vi "Meas Process Record.vi"(5 "result string label":string="str res", 7 "session":T9={"adc"={"niScope"={"channel cfg"=[], "sessions"=[], "multi cards"=FALSE, "channels"=0, "type"=enum."n/a", "memory [B/chn]"=0, "ext. clock [Hz]"=0.0, "samples count"=0, "use streaming"=FALSE, "proc setup"={"packet size [smpl]"=0, "current timeout [s]"=0.0, "blk2blk timeout [s]"=0.0, "event time"=timestamp(0 s since 1904-01-01), "temp sampl T [s]"=0.0, "data queue"=refnum, "stop notifier"=refnum, "proc ref"=refnum}, "sample width [B]"=0, "ranges [V]"=[], "trigger setup"={"coupling"=1, "level [V]"=0.0, "slope"=0, "mode"=enum."Immediate"}, "fs [Hz]"=0.0, "bitres [bit]"=0}, "3458A"={"channels"=[], "sync unit"={"VISA"="", "type"=enum."Picotest U6200A"}, "awg unit"={"type"=enum."Agilent 331xxA to 332xxA", "VISA"="", "enable 10MHz ref"=FALSE}, "sync mode"=enum."MASTER-SLAVE, MASTER clocked by TIMER", "streaming mode"=FALSE, "idn mode"=enum."Auto", "sampling mode"=enum."DCV", "Ts [s]"=0.0, "sample memory [B]"=0, "proc setup"={"channel id"=0, "packet size [smpl]"=0, "current timeout [s]"=0.0, "blk2blk timeout [s]"=0.0, "event time"=timestamp(0 s since 1904-01-01), "stop notifier"=refnum, "data queues"=[], "proc refs"=[], "bus semaphore"=refnum}, "sample size [B]"=0, "sample count"=0, "aux data"={"channel id"=0, "valid?"=[], "gain [V]"=[], "timestamp [s]"=[], "Ts [s]"=0.0, "abs timestamp"=timestamp(0 s since 1904-01-01), "t [deg C]"=[]}, "ranges [V]"=[], "aperture [s]"=0.0, "LEVEL trigger"={"edge"=enum."POS", "level [V]"=0.0, "coupling"=enum."DC"}, "trigger mode"=enum."AUTO", "measure temp.?"=FALSE, "disp mesages"=[], "shared bus?"=FALSE, "disable display?"=FALSE, "aper mode"=enum."Manual", "aper rules"=[]}, "dsdll"={"dsdll"={"dsdll path"=path "", "dsdll handle"=[], "output devices"=[], "capture devices"=[]}, "channels"=0, "device id"=0, "channel idns"=[], "proc setup"={"packet size [smpl]"=0, "current timeout [s]"=0.0, "blk2blk timeout [s]"=0.0, "event time"=timestamp(0 s since 1904-01-01), "data queue"=refnum, "stop notifier"=refnum, "proc ref"=refnum}, "samples count"=0, "fs [Hz]"=0.0}, "type"=enum."niScope", "channel idn str"=[], "aux instr idn str"=[], "modified?"=FALSE, "simadc"={"channels"=[], "range [V]"=0.0, "Ts step [s]"=0.0, "time [s]"=0.0, "fs [Hz]"=0.0, "count"=0, "smpl offset"=0, "set count"=0, "bit res"=0}, "force rst?"=FALSE, "exit mode"=enum."Immediate reset", "exit dly"=0.0, "exit tmr"=timestamp(0 s since 1904-01-01), "busy?"=FALSE, "accessed?"=FALSE, "QuADC session"={"channel cfg"=[], "sessions"=[], "multi cards"=FALSE, "channels"=0, "type"=enum."n/a", "memory [B/chn]"=0, "ext. clock [Hz]"=0.0, "samples count"=0, "use streaming"=FALSE, "proc setup"={"packet size [smpl]"=0, "current timeout [s]"=0.0, "blk2blk timeout [s]"=0.0, "event time"=timestamp(0 s since 1904-01-01), "temp sampl T [s]"=0.0, "data queue"=refnum, "stop notifier"=refnum, "proc ref"=refnum}, "sample width [B]"=0, "ranges [V]"=[], "trigger setup"={"coupling"=1, "level [V]"=0.0, "slope"=0, "mode"=enum."Immediate"}, "fs [Hz]"=0.0, "bitres [bit]"=0}}, "sequence"=[], "sequence setup"={"group setups"=[], "average cycles"=0, "range mode"=enum."Keep defaults", "fs mode"=enum."Frequency", "rng even"=0.0, "rng odd"=0.0, "folder"=path "", "name base"="", "meas id"=0, "settle [s]"=0.0}, "golpi"=refnum, "processing setup"={"mode"=enum."Raw", "call after avgs?"=FALSE, "calculate?"=FALSE, "raw mode"={"command"="", "result mode"=enum."Display console output (only Octave)", "res variable"=""}, "QWTB"={"QWTB path"=path "", "alg filter path"="", "alg ids"=[], "alg parameters"=[], "parsed parameters"=[], "selected alg id"="", "selected unc mode"=enum."None", "qwtb mcc"=100, "qwtb timeout"=90, "qwtb covg"=95.0, "qwtb ofs"=0, "qwtb lim data"=0, "multicore"={"jobs folder"=path "", "cores"=0, "max jobs"=0, "mode"=enum."Singlecore"}, "unc once?"=FALSE}}, "corrections"={"transducers"={"channels"=[], "last path"=path ""}, "digitizer"={"last path"=path "", "channel paths"=[], "channel idns"=[], "correction name"="", "channel names"=[], "folders to copy"=[], "channel valid"=[], "correction path"=path "", "correction rel path"="", "rel folders to copy"=[]}}, "assist cfg"={"P"=0, "Q"=0, "rel shift"=0.0, "ref freq"=0.0, "min fs"=0.0, "max fs tol"=0.0, "min int"=0.0, "max int"=0.0, "max err"=0.0, "max timeout"=0.0}} {"corrections"."transducers"."channels"."Phase index" min=1 step=1; "adc"."QuADC session"."trigger setup"."level [V]" format="%.2f"; "adc"."QuADC session"."trigger setup"."coupling" items=["AC"=0, "DC"=1, "HF Reject"=3, "LF Reject"=4, "AC Plus HF Reject"=1001]; "adc"."QuADC session"."channel cfg"."Clock fr. (Hz)" min=0.0 format="%#_9p"; "adc"."QuADC session"."channel cfg"."Number of JJ" min=1; "adc"."QuADC session"."channel cfg"."Range [Vpk]" min=0.0; "adc"."QuADC session"."channel cfg"."Channel" min=0; "adc"."3458A"."channels"."Range [Vpk]" min=0.0; "adc"."niScope"."trigger setup"."level [V]" format="%.2f"; "adc"."niScope"."trigger setup"."coupling" items=["AC"=0, "DC"=1, "HF Reject"=3, "LF Reject"=4, "AC Plus HF Reject"=1001]; "adc"."niScope"."channel cfg"."Range [Vpk]" min=0.0; "adc"."niScope"."channel cfg"."Channel" min=0}, 8 "error in":errorcluster, 11 "sequence item":T2) -> (0 "error out":errorcluster)   [LabVIEW 2013]
doc: "Processes record defined by sequence item. It executes code defined in 'sequence setup' passed in the 'session'. It executes the command only if calculation is enabled in the sequence setup. Result from Octave console is printed to the named string using SGUI lib."
uses:
  Meas Session.ctl
  adc/ADC Session.ctl
  drivers/niScope/niScope Session.ctl
  drivers/niScope/niScope Virtual Channel Config.ctl
  drivers/niScope/niScope Virtual Channel Mode.ctl
  drivers/niScope/niScope Virtual Channel Input Z.ctl
  drivers/niScope/niScope Virtual Channel Coupling.ctl
  drivers/niScope/niScope Type.ctl
  drivers/niScope/niScope Digitizing Process Options.ctl
  drivers/niScope/niScope Data Packet.ctl
  drivers/niScope/niScope Trigger Setup.ctl
  <instrlib>/niScope/Controls/niScope trigger coupling.ctl
  <instrlib>/niScope/Controls/niScope trigger slope.ctl
  drivers/DMM/3458A Digitizer Session.ctl
  drivers/DMM/3458A Virtual Channel Config.ctl
  drivers/Counter/Counter Session.ctl
  drivers/Counter/Counter Type.ctl
  drivers/AWG/AWG Session.ctl
  drivers/AWG/AWG Type.ctl
  drivers/DMM/3458A Sync Mode.ctl
  drivers/DMM/3458A Idn Mode.ctl
  drivers/DMM/3458A Digitizing Low Levels/Configure/Sampling Mode.ctl
  drivers/DMM/3458A Digitizing Process Options.ctl
  drivers/DMM/3458A Data Packet.ctl
  drivers/DMM/3458A Aux Record Data.ctl
  drivers/DMM/3458A Digitizing Low Levels/Configure/Level Setup.ctl
  drivers/DMM/3458A Digitizing Low Levels/Configure/First Sample Trigger.ctl
  drivers/DMM/3458A Aperture Selection Mode.ctl
  drivers/dsdll/DSDLL Session.ctl
  drivers/dsdll/dsdll.lvlibp/dsdll_instance.ctl
  drivers/dsdll/dsdll.lvlibp/dsdll_device_record.ctl
  drivers/dsdll/DSDLL Process Config.ctl
  drivers/dsdll/DSDLL Data Packet.ctl
  adc/ADC Type.ctl
  drivers/simulated_adc/SimAdc Config.ctl
  drivers/simulated_adc/SimAdc Channel Cfg.ctl
  adc/ADC On Close Action.ctl
  drivers/Quatsch_driver/QuADCDriver/QuADC Session.ctl
  drivers/Quatsch_driver/QuADCDriver/QuADC Virtual Channel Config.ctl
  drivers/Quatsch_driver/QuADCDriver/QuADC Virtual Channel Mode.ctl
  drivers/Quatsch_driver/QuADCDriver/QuADC Virtual Channel Input Z.ctl
  drivers/Quatsch_driver/QuADCDriver/QuADC Virtual Channel Coupling.ctl
  drivers/Quatsch_driver/QuADCDriver/QuADC Type.ctl
  drivers/Quatsch_driver/QuADCDriver/QuADC Digitizing Process Options.ctl
  drivers/Quatsch_driver/QuADCDriver/QuADC Data Packet.ctl
  drivers/Quatsch_driver/QuADCDriver/QuADC Trigger Setup.ctl
  Meas Sequence Item.ctl
  Meas Sampling Configuration.ctl
  adc/ADC Trig Config.ctl
  adc/ADC Trig Mode Source.ctl
  adc/ADC Trig Coupling.ctl
  adc/ADC Trig Slope.ctl
  QWTB/Meas Proc QWTB Algorithm Parameter Data.ctl
  Meas Sequence Configuration.ctl
  Meas Range Mode.ctl
  Meas Sampling Rate Mode.ctl
  octave/golpi/mpc/golpi_session_ref.ctl
  octave/golpi/mpc/golpi_session.ctl
  octave/golpi/GOLPI Library.lvlibp/Public/GOLPI reference Type Def.ctl
  octave/golpi/GOLPI Library.lvlibp/LV Process source distribution/Pipe Handle.ctl
  Meas Process Config.ctl
  Meas Process Mode.ctl
  Meas Process Raw Config.ctl
  Meas Process Raw Result Mode.ctl
  QWTB/Meas Proc QWTB Setup.ctl
  QWTB/Meas Proc QWTB Uncertainty Mode.ctl
  QWTB/Meas Proc QWTB Multicore Setup.ctl
  QWTB/Meas Proc QWTB Multicore Type.ctl
  Corrections/Corr Setup.ctl
  Corrections/Corr Tranducer Item.ctl
  Corrections/Corr Digitizers.ctl
  Assist/Assist Panel Setup.ctl
  varilib/SGUI Assign Multiple Strings With Tags By Label.vi
  octave/golpi/GOLPI Library.lvlibp/Private/Get Variable - polymorph parts/Get String.vi
  varilib/varilib.lvlib
  octave/golpi/mpc/GOLPI Multi Process.lvlib
  octave/golpi/GOLPI Library.lvlibp
  drivers/niScope/niScope Virtual Digitizer.lvlib
  drivers/DMM/3458A Virtual Digitizer.lvlib
  drivers/Counter/Counter.lvlib
  drivers/AWG/AWG.lvlib
  drivers/DMM/3458A Digitizing Low Levels/3458A Digitizing Low Levels.lvlib
  drivers/dsdll/dsdll.lvlibp
  drivers/dsdll/DSDLL Virtual Digitizer.lvlib
  octave/golpi/GOLPI Library.lvlibp/LV Process source distribution/LV Process library.lvlib
  drivers/Quatsch_driver/QuADCDriver/QuADC Virtual Digitizer.lvlib
panel:
  in  "mode":T1
  # "ADC:"
  # "IP Address"
  # "."
  # "."
  # "."
  # ":"
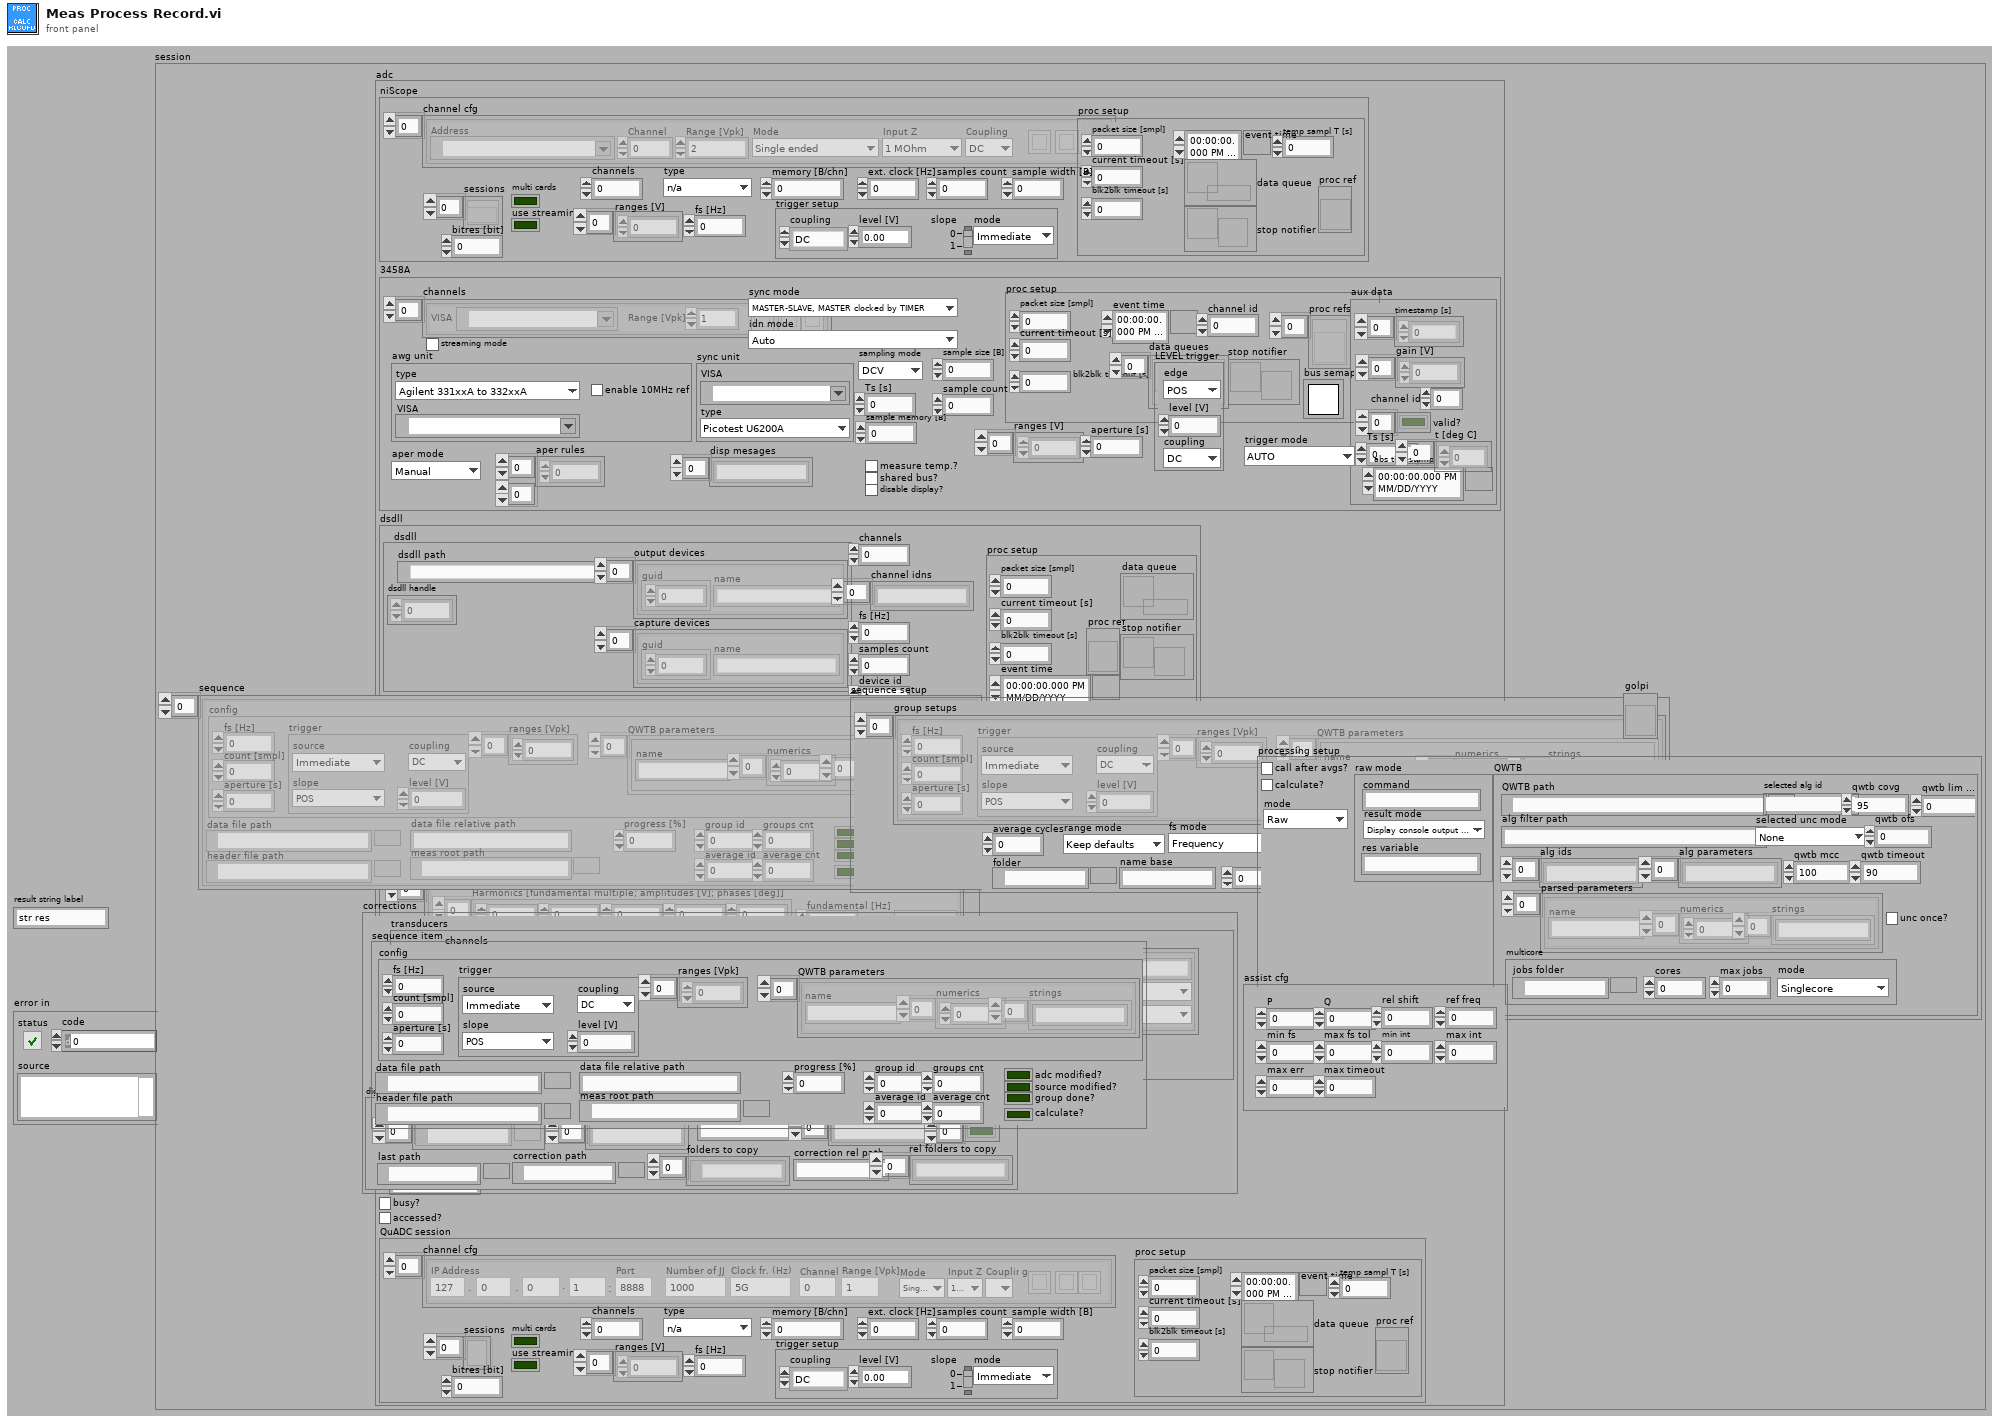
[diagram p1: front panel]
types:
  T1 = typedef "Meas Proc QWTB Multicore Type.ctl" = enum16{"Singlecore", "Multicore", "Multistation"}
  T2 = typedef "Meas Sequence Item.ctl" = cluster{"config":T3, "data file path":path, "header file path":path, "group id":i32, "average id":i32, "group done?":bool, "adc modified?":bool, "source modified?":bool, "progress [%]":dbl, "groups cnt":i32, "average cnt":i32, "data file relative path":string, "meas root path":path, "calculate?":bool}
  T3 = typedef "Meas Sampling Configuration.ctl" = cluster{"fs [Hz]":dbl, "count [smpl]":i64, "aperture [s]":dbl, "trigger":T4, "ranges [Vpk]":dbl[], "QWTB parameters":T8[]}
  T4 = typedef "ADC Trig Config.ctl" = cluster{"source":T5, "level [V]":dbl, "coupling":T6, "slope":T7}
  T5 = typedef "ADC Trig Mode Source.ctl" = enum16{"Immediate", "External", "Level"}
  T6 = typedef "ADC Trig Coupling.ctl" = enum16{"DC", "AC"}
  T7 = typedef "ADC Trig Slope.ctl" = enum16{"POS", "NEG"}
  T8 = typedef "Meas Proc QWTB Algorithm Parameter Data.ctl" = cluster{"name":string, "numerics":dbl[], "strings":string[]}
  T9 = typedef "Meas Session.ctl" = cluster{"adc":T10, "sequence":T2[], "sequence setup":T52, "golpi":T55, "processing setup":T56, "corrections":T63, "assist cfg":T66}
  T10 = typedef "ADC Session.ctl" = cluster{"niScope":T11, "3458A":T21, "dsdll":T36, "type":T40, "channel idn str":string[], "aux instr idn str":string[], "modified?":bool, "simadc":T41, "force rst?":bool, "exit mode":T43, "exit dly":dbl, "exit tmr":timestamp, "busy?":bool, "accessed?":bool, "QuADC session":T44}
  T11 = typedef "niScope Virtual Digitizer.lvlib/niScope Session.ctl" = cluster{"channel cfg":T12[], "sessions":refnum<k20>[], "multi cards":bool, "channels":i32, "type":T16, "memory [B/chn]":i32, "ext. clock [Hz]":dbl, "samples count":i64, "use streaming":bool, "proc setup":T17, "sample width [B]":i32, "ranges [V]":dbl[], "trigger setup":T18, "fs [Hz]":dbl, "bitres [bit]":i32}
  T12 = typedef "niScope Virtual Digitizer.lvlib/niScope Virtual Channel Config.ctl" = cluster{"Address":refnum<k15>, "Channel":i32, "Mode":T13, "Input Z":T14, "Coupling":T15, "Range [Vpk]":dbl, "btn clr":bool, "btn up":bool, "btn down":bool}
  T13 = typedef "niScope Virtual Digitizer.lvlib/niScope Virtual Channel Mode.ctl" = enum16{"Single ended", "Unbal. differential", "Differential"}
  T14 = typedef "niScope Virtual Digitizer.lvlib/niScope Virtual Channel Input Z.ctl" = enum16{"1 MOhm", "50 Ohm"}
  T15 = typedef "niScope Virtual Digitizer.lvlib/niScope Virtual Channel Coupling.ctl" = enum16{"AC", "DC", "GND"}
  T16 = typedef "niScope Virtual Digitizer.lvlib/niScope Type.ctl" = enum16{"n/a", "5922"}
  T17 = typedef "niScope Virtual Digitizer.lvlib/niScope Digitizing Process Options.ctl" = cluster{"packet size [smpl]":i64, "current timeout [s]":dbl, "blk2blk timeout [s]":dbl, "event time":timestamp, "temp sampl T [s]":dbl, "data queue":refnum<queue>, "stop notifier":refnum<notifier>, "proc ref":refnum<vi>}
  T18 = typedef "niScope Virtual Digitizer.lvlib/niScope Trigger Setup.ctl" = cluster{"coupling":T19, "level [V]":dbl, "slope":T20, "mode":enum16{"Immediate", "External", "Level"}}
  T19 = typedef "niScope trigger coupling.ctl" = u16
  T20 = typedef "niScope trigger slope.ctl" = i32
  T21 = typedef "3458A Virtual Digitizer.lvlib/3458A Digitizer Session.ctl" = cluster{"channels":T22[], "sync unit":T23, "awg unit":T25, "sync mode":T27, "streaming mode":bool, "idn mode":T28, "sampling mode":T29, "Ts [s]":dbl, "sample memory [B]":i32, "proc setup":T30, "sample size [B]":i32, "sample count":i32, "aux data":T32, "ranges [V]":dbl[], "aperture [s]":dbl, "LEVEL trigger":T33, "trigger mode":T34, "measure temp.?":bool, "disp mesages":string[], "shared bus?":bool, "disable display?":bool, "aper mode":T35, "aper rules":dbl[][]}
  T22 = typedef "3458A Virtual Digitizer.lvlib/3458A Virtual Channel Config.ctl" = cluster{"VISA":refnum<visa-resource-name>, "Range [Vpk]":dbl, "btn clr":bool, "btn up":bool, "btn down":bool}
  T23 = typedef "Counter.lvlib/Counter Session.ctl" = cluster{"VISA":refnum<visa-resource-name>, "type":T24}
  T24 = typedef "Counter.lvlib/Counter Type.ctl" = enum16{"Picotest U6200A", "dummy"}
  T25 = typedef "AWG.lvlib/AWG Session.ctl" = cluster{"type":T26, "VISA":refnum<visa-resource-name>, "enable 10MHz ref":bool}
  T26 = typedef "AWG.lvlib/AWG Type.ctl" = enum16{"Agilent 331xxA to 332xxA", "Agilent 335xxA to 336xxA", "Tektronix AFG3101C", "dummy"}
  T27 = typedef "3458A Virtual Digitizer.lvlib/3458A Sync Mode.ctl" = enum16{"MASTER-SLAVE, MASTER clocked by TIMER", "MASTER-SLAVE, MASTER clocked by AWG", "ALL clocked by AWG", "MASTER-SLAVE, ALL clocked by TIMER", "ALL clocked by AWG with DFLL"}
  T28 = typedef "3458A Virtual Digitizer.lvlib/3458A Idn Mode.ctl" = enum16{"Auto", "Sequential (chn A, chn B, ...)", "From calibration string"}
  T29 = typedef "3458A Virtual Digitizer.lvlib/3458A Digitizing Low Levels.lvlib/Sampling Mode.ctl" = enum16{"DCV", "DSDC", "DSAC"}
  T30 = typedef "3458A Virtual Digitizer.lvlib/3458A Digitizing Process Options.ctl" = cluster{"channel id":i32, "packet size [smpl]":i32, "current timeout [s]":dbl, "blk2blk timeout [s]":dbl, "event time":timestamp, "stop notifier":refnum<notifier>, "data queues":refnum<queue>[], "proc refs":refnum<vi>[], "bus semaphore":T31}
  T31 = typedef "Semaphore RefNum" = refnum<k1>
  T32 = typedef "3458A Virtual Digitizer.lvlib/3458A Aux Record Data.ctl" = cluster{"channel id":i32, "valid?":bool[], "gain [V]":dbl[], "timestamp [s]":dbl[], "Ts [s]":dbl, "abs timestamp":timestamp, "t [deg C]":dbl[]}
  T33 = typedef "3458A Virtual Digitizer.lvlib/3458A Digitizing Low Levels.lvlib/Level Setup.ctl" = cluster{"edge":enum16{"POS", "NEG"}, "level [V]":dbl, "coupling":enum16{"DC", "AC"}}
  T34 = typedef "3458A Virtual Digitizer.lvlib/3458A Digitizing Low Levels.lvlib/First Sample Trigger.ctl" = enum16{"AUTO", "EXT", "SYN", "SGL", "HOLD", "LEVEL"}
  T35 = typedef "3458A Virtual Digitizer.lvlib/3458A Aperture Selection Mode.ctl" = enum16{"Manual", "Maximum", "Table"}
  T36 = typedef "DSDLL Virtual Digitizer.lvlib/DSDLL Session.ctl" = cluster{"dsdll":T37, "channels":i32, "device id":i32, "channel idns":string[], "proc setup":T39, "samples count":i32, "fs [Hz]":dbl}
  T37 = typedef "dsdll.lvlibp/dsdll_instance.ctl" = cluster{"dsdll path":path, "dsdll handle":u8[], "output devices":T38[], "capture devices":T38[]}
  T38 = typedef "dsdll.lvlibp/dsdll_device_record.ctl" = cluster{"guid":u8[], "name":string}
  T39 = typedef "DSDLL Virtual Digitizer.lvlib/DSDLL Process Config.ctl" = cluster{"packet size [smpl]":i32, "current timeout [s]":dbl, "blk2blk timeout [s]":dbl, "event time":timestamp, "data queue":refnum<queue>, "stop notifier":refnum<notifier>, "proc ref":refnum<vi>}
  T40 = typedef "ADC Type.ctl" = enum16{"niScope", "3458A", "DirectSound DLL", "dummy", "QuADC"}
  T41 = typedef "SimAdc Config.ctl" = cluster{"channels":T42[], "range [V]":dbl, "Ts step [s]":dbl, "time [s]":dbl, "fs [Hz]":dbl, "count":i64, "smpl offset":i64, "set count":i64, "bit res":i32}
  T42 = typedef "SimAdc Channel Cfg.ctl" = cluster{"harmonics":dbl[][], "btn clear":bool, "noise":dbl, "fundamental [Hz]":dbl}
  T43 = typedef "ADC On Close Action.ctl" = enum16{"Immediate reset", "Delayed reset"}
  T44 = typedef "QuADC Virtual Digitizer.lvlib/QuADC Session.ctl" = cluster{"channel cfg":T45[], "sessions":refnum<k5>[], "multi cards":bool, "channels":i32, "type":T49, "memory [B/chn]":i32, "ext. clock [Hz]":dbl, "samples count":i64, "use streaming":bool, "proc setup":T50, "sample width [B]":i32, "ranges [V]":dbl[], "trigger setup":T51, "fs [Hz]":dbl, "bitres [bit]":i32}
  T45 = typedef "QuADC Virtual Digitizer.lvlib/QuADC Virtual Channel Config.ctl" = cluster{"Channel":i32, "Mode":T46, "Input Z":T47, "Coupling":T48, "Range [Vpk]":dbl, "btn clr":bool, "btn up":bool, "btn down":bool, "IP address A":u8, "IP address B":u8, "IP address C":u8, "IP address D":u8, "Port":u16, "Number of JJ":u32, "Clock fr. (Hz)":dbl}
  T46 = typedef "QuADC Virtual Digitizer.lvlib/QuADC Virtual Channel Mode.ctl" = enum16{"Single ended", "Unbal. differential", "Differential"}
  T47 = typedef "QuADC Virtual Digitizer.lvlib/QuADC Virtual Channel Input Z.ctl" = enum16{"1 MOhm", "50 Ohm"}
  T48 = typedef "QuADC Virtual Digitizer.lvlib/QuADC Virtual Channel Coupling.ctl" = enum16{"AC", "DC", "GND"}
  T49 = typedef "QuADC Virtual Digitizer.lvlib/QuADC Type.ctl" = enum16{"n/a", "v1"}
  T50 = typedef "QuADC Virtual Digitizer.lvlib/QuADC Digitizing Process Options.ctl" = cluster{"packet size [smpl]":i64, "current timeout [s]":dbl, "blk2blk timeout [s]":dbl, "event time":timestamp, "temp sampl T [s]":dbl, "data queue":refnum<queue>, "stop notifier":refnum<notifier>, "proc ref":refnum<vi>}
  T51 = typedef "QuADC Virtual Digitizer.lvlib/QuADC Trigger Setup.ctl" = cluster{"coupling":T19, "level [V]":dbl, "slope":T20, "mode":enum16{"Immediate", "External", "Level"}}
  T52 = typedef "Meas Sequence Configuration.ctl" = cluster{"group setups":T3[], "average cycles":i32, "range mode":T53, "fs mode":T54, "rng even":dbl, "rng odd":dbl, "folder":path, "name base":string, "meas id":i32, "settle [s]":dbl}
  T53 = typedef "Meas Range Mode.ctl" = enum16{"Keep defaults", "Set All channels", "Set Odd and Even channels"}
  T54 = typedef "Meas Sampling Rate Mode.ctl" = enum16{"Frequency", "Period"}
  T55 = typedef "GOLPI Multi Process.lvlib/golpi_session_ref.ctl" = refnum<vi>
  T56 = typedef "Meas Process Config.ctl" = cluster{"mode":T57, "call after avgs?":bool, "calculate?":bool, "raw mode":T58, "QWTB":T60}
  T57 = typedef "Meas Process Mode.ctl" = enum16{"Raw", "QWTB"}
  T58 = typedef "Meas Process Raw Config.ctl" = cluster{"command":string, "result mode":T59, "res variable":string}
  T59 = typedef "Meas Process Raw Result Mode.ctl" = enum16{"Display console output (only Octave)", "Display string variable", "Display result file %respath%"}
  T60 = typedef "Meas Proc QWTB Setup.ctl" = cluster{"QWTB path":path, "alg filter path":string, "alg ids":string[], "alg parameters":string[], "parsed parameters":T8[], "selected alg id":string, "selected unc mode":T61, "qwtb mcc":i32, "qwtb timeout":i32, "qwtb covg":dbl, "qwtb ofs":i64, "qwtb lim data":i64, "multicore":T62, "unc once?":bool}
  T61 = typedef "Meas Proc QWTB Uncertainty Mode.ctl" = enum16{"None", "GUF", "Monte Carlo"}
  T62 = typedef "Meas Proc QWTB Multicore Setup.ctl" = cluster{"jobs folder":path, "cores":i32, "max jobs":i32, "mode":T1}
  T63 = typedef "Corr Setup.ctl" = cluster{"transducers":cluster{"channels":T64[], "last path":path}, "digitizer":T65}
  T64 = typedef "Corr Tranducer Item.ctl" = cluster{"Path":path, "Ratio:":string, "Name:":string, "btn rem":bool, "btn up":bool, "btn down":bool, "s.n.:":string, "btn open":bool, "ratio o/i":dbl, "chn hi":u16, "chn lo":u16, "Phase index":i32}
  T65 = typedef "Corr Digitizers.ctl" = cluster{"last path":path, "channel paths":path[], "channel idns":string[], "correction name":string, "channel names":string[], "folders to copy":path[], "channel valid":bool[], "correction path":path, "correction rel path":string, "rel folders to copy":string[]}
  T66 = typedef "Assist Panel Setup.ctl" = cluster{"P":i32, "Q":i32, "rel shift":dbl, "ref freq":dbl, "min fs":dbl, "max fs tol":dbl, "min int":dbl, "max int":dbl, "max err":dbl, "max timeout":dbl}
  T67 = typedef "GOLPI Library.lvlibp/GOLPI reference Type Def.ctl" = cluster{"pipe handle":T68, "fast read timeout [ms]":u32, "fast read settle time [ms]":u32, "fast read to multiple [ms]":u32, "max elements per input line":u32, "slow read timeout [ms]":u32, "stdin double format specifier":string, "max elements per stdout output column":u32, "console mode bitstream":bool, "bitstream first read timeout [ms]":u32, "bitstream read timeout [ms]":u32, "struct transfer possible":bool, "matlab mode":bool}
  T68 = typedef "GOLPI Library.lvlibp/LV Process library.lvlib/Pipe Handle.ctl" = cluster{"lv_proc.dll file path":path, "process instance handle":u32[], "debug mode":bool, "debug data":cluster{"time":timestamp, "stdin":bool, "data":string}[]}
  T69 = typedef "GOLPI Multi Process.lvlib/golpi_session.ctl" = cluster{"GOLPI ref":T67, "idn str":string, "octave path":path, "work path":path, "start timeout [ms]":u32, "clr cache":bool, "console":bool, "binary":bool, "semaphore":T31, "initial command":string, "exit command":string, "matlab":bool}
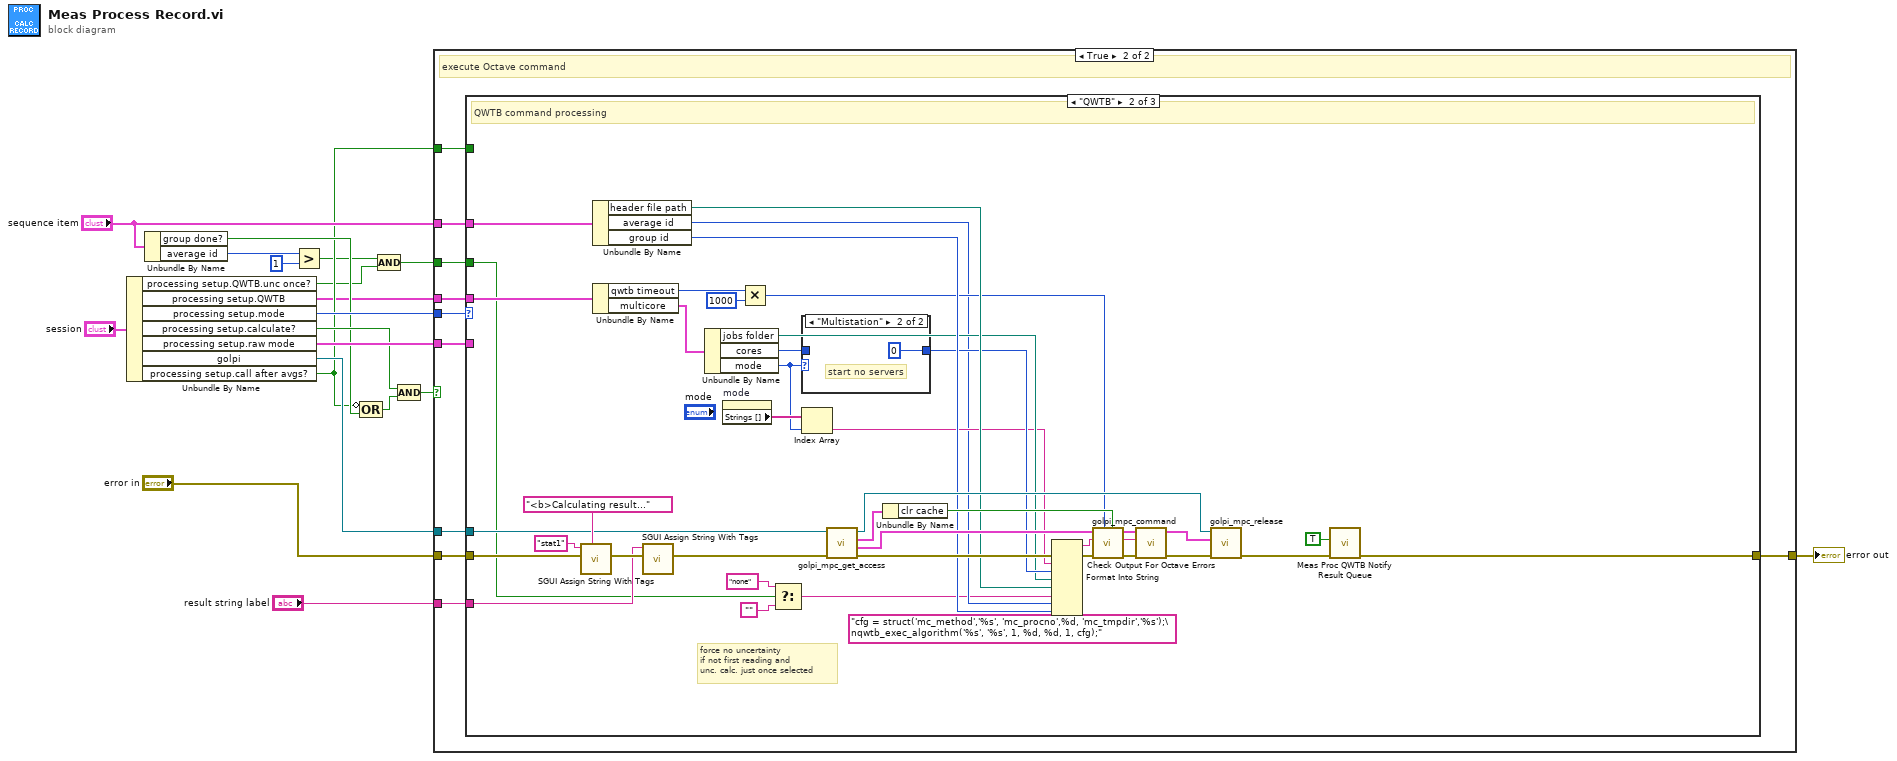
[diagram p0: block diagram]
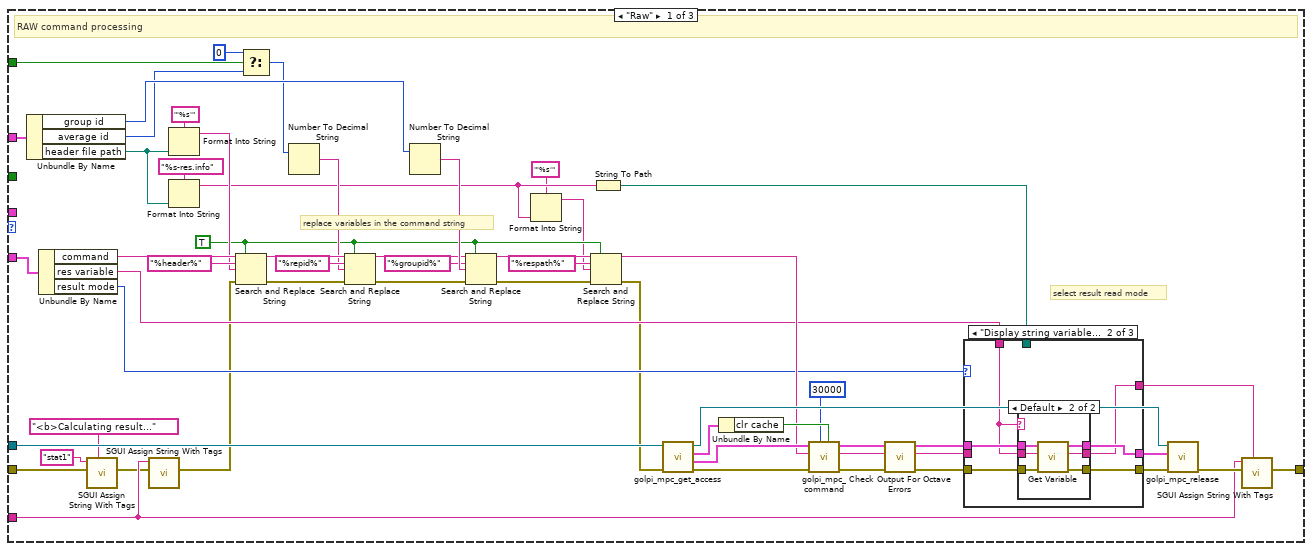
[diagram p3: hidden frame]
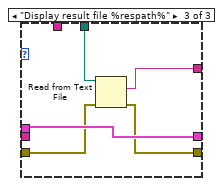
[diagram p6: hidden frame]
diagram:
  n1 = Unbundle By Name("session") -> ("processing setup.QWTB.unc once?"=w4:bool, "processing setup.QWTB"=w6:T60, "processing setup.mode"=w13:T57, "processing setup.calculate?"=w11:bool, "processing setup.raw mode"=w14:T58, "golpi"=w17:T55, "processing setup.call after avgs?"=w7:bool)
  n2 = Unbundle By Name("sequence item") -> ("group done?"=w8:bool, "average id"=w2:i32)
  n3 = Greater?(x=w2, y=1) -> (0:w5:bool)
  n4 = Compound Arithmetic op=OR(invert w7, w8) -> (w10:bool)
  n5 = Compound Arithmetic op=AND(w5, w4) -> (w3:bool)
  n6 = Compound Arithmetic op=AND(w11, w10) -> (w12:bool)
  n7 = case shown="True" w12 {
    tunnel: "error in" -> [w20 w27]
    tunnel: w17 -> [_ w30]
    tunnel: [w20 w29] -> w16
    tunnel: "result string label" -> [_ w28]
    tunnel: w14 -> [_ w26]
    tunnel: "sequence item" -> [_ w25]
    tunnel: w13 -> [_ w24]
    tunnel: w7 -> [_ w23]
    tunnel: w6 -> [_ w22]
    tunnel: w3 -> [_ w21]
    frame False {
    }
    frame True {
      # "execute Octave command"
      n8 = case shown="\"QWTB\"" w24 {
        tunnel: w30 -> [w84 w131 _]
        tunnel: [w78 w128 w151] -> w29
        tunnel: w28 -> [w75 w133 _]
        tunnel: w27 -> [w73 w135 w151]
        tunnel: w26 -> [w70 _ _]
        tunnel: w25 -> [w62 w143 _]
        tunnel: w23 -> [w40 _ _]
        tunnel: w22 -> [_ w130 _]
        tunnel: w21 -> [_ w110 _]
        frame "Raw" {
          w51 = TRUE ("replace all? (F)")
          # "select result read mode"
          # "replace variables in the command string"
          # "RAW command processing"
          n9 = Unbundle By Name(w62) -> ("group id"=w55:i32, "average id"=w39:i32, "header file path"=w65:path)
          n10 = Unbundle By Name(w70) -> ("command"=w69:string, "res variable"=w46:string, "result mode"=w45:T59)
          n11 = call-poly "SGUI Assign String With Tags.vi"("error in"=w73, "label(s) (empty)"="stat1", "string (empty)"="<b>Calculating result...") -> ("error out"=w74:errorcluster)  [unwired: 7 in, 1 out]
          n12 = call-poly "SGUI Assign String With Tags.vi"("error in"=w74, "label(s) (empty)"=w75) -> ("error out"=w41:errorcluster)  [unwired: 8 in, 1 out]
          n13 = Format Into String(format string="'%s'", w65) -> (resulting string=w61:string)  [unwired: 2 in, 1 out]
          n14 = Format Into String(format string="%s-res.info", w65) -> (resulting string=w35:string)  [unwired: 2 in, 1 out]
          n15 = Search and Replace String(replace all?=w51, input string=w69, search string="%header%", replace string=w61, error in=w41) -> (result string=w68:string, error out=w66:errorcluster)  [unwired: 3 in, 2 out]
          n16 = Select(t=0, s=w40, f=w39) -> (s? t:f=w38:i32)
          n17 = Number To Decimal String(number=w38) -> (decimal integer string=w60:string)  [unwired: 1 in]
          n18 = Search and Replace String(replace all?=w51, input string=w68, search string="%repid%", replace string=w60, error in=w66) -> (result string=w56:string, error out=w57:errorcluster)  [unwired: 3 in, 2 out]
          n19 = Number To Decimal String(number=w55) -> (decimal integer string=w59:string)  [unwired: 1 in]
          n20 = Search and Replace String(replace all?=w51, input string=w56, search string="%groupid%", replace string=w59, error in=w57) -> (result string=w52:string, error out=w53:errorcluster)  [unwired: 3 in, 2 out]
          n21 = Format Into String(format string="'%s'", w35) -> (resulting string=w36:string)  [unwired: 2 in, 1 out]
          n22 = Search and Replace String(replace all?=w51, input string=w52, search string="%respath%", replace string=w36, error in=w53) -> (result string=w50:string, error out=w42:errorcluster)  [unwired: 3 in, 2 out]
          n23 = String To Path(string=w35) -> (path=w44:path)
          n24 = call "golpi_mpc_get_access.vi"("error in"=w42, "golpi session ref"=w84) -> ("error out"=w85:errorcluster, "GOLPI ref out"=w83:T67, "golpi session out"=w82:T69, "golpi session ref out (copy)"=w80:T55)  [unwired: 4 in, 2 out]
          n25 = Unbundle By Name(w82) -> ("clr cache"=w81:bool)
          n26 = call "golpi_mpc_command.vi"("clear function cache before command? (False)"=w81, "timeout [ms]"=u32 30000, "error in"=w85, "command"=w50, "GOLPI ref in"=w83) -> ("error out"=w33:errorcluster, "read buffer"=w32:string, "GOLPI ref. out"=w49:T67)  [unwired: 4 in]
          n27 = call "Check Output For Octave Errors.vi"("error in"=w33, "read buffer"=w32) -> ("error out"=w31:errorcluster)  [unwired: 9 in]
          n28 = case shown="\"Display string variable\"" w45 {
            tunnel: w31 -> [w86 w94 w106]
            tunnel: w49 -> [w87 w93 w107]
            tunnel: [w86 w92 w105] -> w48
            tunnel: [w87 w91 w107] -> w47
            tunnel: w46 -> [_ w89 _]
            tunnel: [w88 w90 w103] -> w43
            tunnel: w32 -> [w88 _ _]
            tunnel: w44 -> [_ _ w104]
            frame "Display console output (only Octave)", Default {
            }
            frame "Display string variable" {
              n29 = case shown="Default" w89 {
                tunnel: w94 -> [w96 w102]
                tunnel: w93 -> [w95 w101]
                tunnel: [w96 w100] -> w92
                tunnel: [w95 w99] -> w91
                tunnel: w89 -> [_ w98]
                tunnel: [_ w97] -> w90
                frame "" {
                }
                frame Default {
                  n30 = call-poly "Get Variable.vi"("error in"=w102, "variable name"=w98, "GOLPI ref. in"=w101) -> ("error out"=w100:errorcluster, "value"=w97:string, "GOLPI ref. out"=w99:T67)  [unwired: 6 in]
                }
              }
            }
            frame "Display result file %respath%" {
              n31 = Read from Text File(file (use dialog)=w104, error in=w106) -> (text=w103:string, error out=w105:errorcluster)  [unwired: 2 in, 2 out]
            }
          }
          n32 = call "golpi_mpc_release.vi"("error in"=w48, "golpi ref or golpi session in"=w47, "golpi session ref"=w80) -> ("error out"=w79:errorcluster)  [unwired: 7 in, 1 out]
          n33 = call-poly "SGUI Assign String With Tags.vi"("error in"=w79, "label(s) (empty)"=w75, "string (empty)"=w43) -> ("error out"=w78:errorcluster)  [unwired: 7 in, 1 out]
        }
        frame "QWTB" {
          # "force no uncertainty\nif not first reading and\nunc. calc. just once selected"
          # "QWTB command processing"
          n34 = call-poly "SGUI Assign String With Tags.vi"("error in"=w135, "label(s) (empty)"="stat1", "string (empty)"="<b>Calculating result...") -> ("error out"=w138:errorcluster)  [unwired: 7 in, 1 out]
          n35 = Unbundle By Name(w143) -> ("header file path"=w132:path, "average id"=w112:i32, "group id"=w123:i32)
          n36 = Unbundle By Name(w130) -> ("qwtb timeout"=w122:i32, "multicore"=w119:T62)
          n37 = call-poly "SGUI Assign String With Tags.vi"("error in"=w138, "label(s) (empty)"=w133) -> ("error out"=w134:errorcluster)  [unwired: 8 in, 1 out]
          n38 = Unbundle By Name(w119) -> ("jobs folder"=w116:path, "cores"=w118:i32, "mode"=w114:T1)
          n39 = property on="mode" class="Enum (strict)"() -> ("Strings []"=w115:string[])  [unwired: 2 in, 2 out]
          n40 = Multiply(x=w122, y=1000) -> (x*y=w120:i32)
          n41 = Select(t="none", s=w110, f="") -> (s? t:f=w111:string)
          n42 = case shown="\"Multistation\"" w114 {
            tunnel: [w149 0 ("cores")] -> w117
            tunnel: w118 -> [w149 _]
            frame Default {
            }
            frame "Multistation" {
              # "start no servers"
            }
          }
          n43 = Index Array(array=w115, index=w114) -> (element=w113:string)
          n44 = call "golpi_mpc_get_access.vi"("error in"=w134, "golpi session ref"=w131) -> ("error out"=w141:errorcluster, "GOLPI ref out"=w148:T67, "golpi session out"=w147:T69, "golpi session ref out (copy)"=w145:T55)  [unwired: 4 in, 2 out]
          n45 = Unbundle By Name(w147) -> ("clr cache"=w146:bool)
          n46 = Format Into String(format string="cfg = struct('mc_method','%s', 'mc_procno',%d, 'mc_tmpdir','%s');\nqwtb_exec_algorithm('%s', '%s', 1, %d, %d, 1, cfg);", error in=w141, w113, w117, w116, w132, w111, w112, w123) -> (resulting string=w140:string, error out=w142:errorcluster)  [unwired: 1 in]
          n47 = call "golpi_mpc_command.vi"("clear function cache before command? (False)"=w146, "timeout [ms]"=w120, "error in"=w142, "command"=w140, "GOLPI ref in"=w148) -> ("error out"=w126:errorcluster, "read buffer"=w124:string, "GOLPI ref. out"=w144:T67)  [unwired: 4 in]
          n48 = call "Check Output For Octave Errors.vi"("error in"=w126, "read buffer"=w124) -> ("error out"=w125:errorcluster)  [unwired: 9 in]
          n49 = call "golpi_mpc_release.vi"("error in"=w125, "golpi ref or golpi session in"=w144, "golpi session ref"=w145) -> ("error out"=w129:errorcluster)  [unwired: 7 in, 1 out]
          n50 = call "Meas Proc QWTB Notify Result Queue.vi"("error in"=w129, "new result? (False)"=TRUE) -> ("error out"=w128:errorcluster)  [unwired: 8 in, 1 out]
        }
        frame Default {
        }
      }
    }
  }
  "error out" <- w16
